vi "GetOperationError.vi"(10 "Additional Information":string, 11 "Operation Error Type":T1) -> (0 "error out":errorcluster)   [LabVIEW 2014]
uses:
  OperationErrorType.ctl
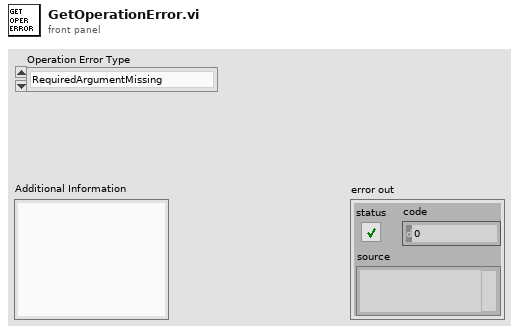
[diagram p1: front panel]
types:
  T1 = typedef "OperationErrorType.ctl" = enum16{"RequiredArgumentMissing", "UnknownArguments", "LoggerSetMultipleTimes", "OperationBrokenError"}
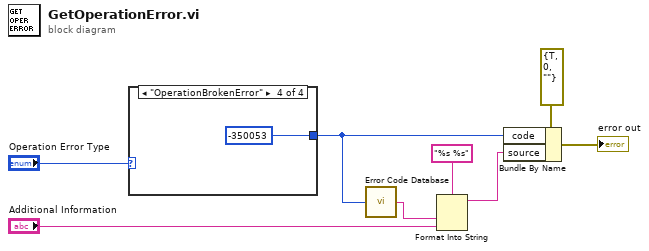
[diagram p0: block diagram]
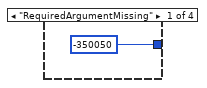
[diagram p2: hidden frame]
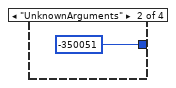
[diagram p3: hidden frame]
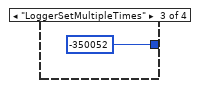
[diagram p4: hidden frame]
diagram:
  n1 = case shown="\"OperationBrokenError\"" "Operation Error Type" {
    tunnel: [-350050 ("code") -350051 ("code") -350052 ("code") -350053 ("code")] -> w2
    frame "RequiredArgumentMissing" {
    }
    frame "UnknownArguments" {
    }
    frame "LoggerSetMultipleTimes" {
    }
    frame "OperationBrokenError" {
    }
  }
  n2 = call <vilib>:"Error Code Database.vi"("Error Code"=w2) -> ("Error Text"=w1:string)
  n3 = Format Into String(format string="%s %s", w1, "Additional Information") -> (resulting string=w4:string)  [unwired: 2 in, 1 out]
  n4 = Bundle By Name(cluster=errorcluster {"status"=TRUE, "code"=0, "source"=""} ("error constant"), "code"=w2, "source"=w4) -> (→"error out":errorcluster)
